vi "FalseTest.vi"() -> ()   [LabVIEW 2016, in "test_AssertControlValue.lvlib"]
uses:
  test_AssertControlValue.lvlib
  main/apis/Setup/GetVI/GetVIByPath.vi
  main/apis/Stimulus/ValueSignal/ValueSignalByPathString.vi
  main/apis/Assert/AssertControlValue/False.vi
  main/apis/Assert/AssertControlValue/Greater.vi
  main/apis/Setup/GetVI/GetVI.lvlib
  <vilib>/addons/_JKI Toolkits/Caraya/classes/Test/Test.lvclass
  main/apis/Assert/AssertControlValue/AssertControlValue.lvlib
panel:
  out "error out":errorcluster
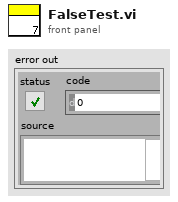
[diagram p1: front panel]
types:
  T1 = enum32{"Invalid", "Standard", "Closed", "Hidden", "Minimized", "Maximized"}
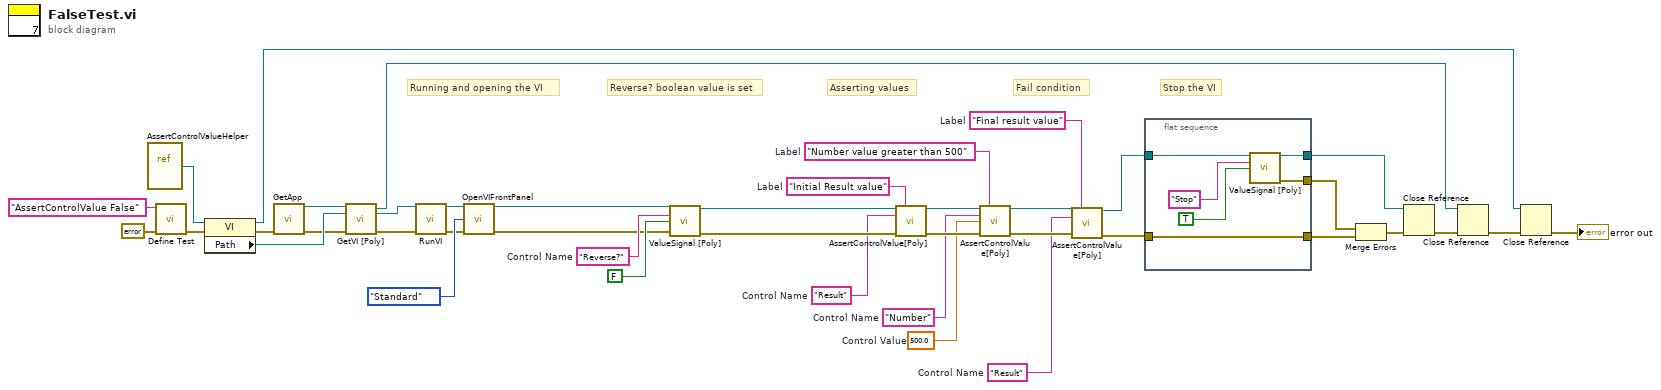
[diagram p0: block diagram]
diagram:
  w5 = "Result"  # Control Name
  w6 = "Final result value"  # Label
  w8 = "Number value greater than 500"  # Label
  w9 = 500.0  # Control Value
  w10 = "Number"  # Control Name
  w16 = "Initial Result value"  # Label
  w27 = "Result"  # Control Name
  w37 = "Reverse?"  # Control Name
  # "Stop the VI"
  # "Asserting values"
  # "Reverse? boolean value is set"
  # "Running and opening the VI"
  # "Fail condition"
  n1 = vi-ref "AssertControlValueHelper.vi"() -> (w31:refnum<vi>)
  n2 = call <vilib>:"Define Test.vi"("error in (no error)"=errorcluster {"status"=FALSE, "code"=0, "source"=""}, "Label (VI Title)"="AssertControlValue False") -> ("error out"=w32:errorcluster)  [unwired: 9 in]
  n3 = property on="Property Node" class="VI"(reference=w31, error in=w32) -> (reference out=w1:refnum<vi>, error out=w40:errorcluster, "Path"=w39:path)
  n4 = call "GetApp.vi"("error in (no error)"=w40) -> ("Application Ref"=w41:refnum<vi>, "error out"=w38:errorcluster)  [unwired: 13 in]
  n5 = call-poly "GetVI [Poly].vi"("Application Ref in"=w41, "VI Path"=w39, "error in (no error)"=w38) -> ("Application Ref out"=w2:refnum<vi>, "VI Reference"=w35:refnum<vi>, "error out"=w34:errorcluster)  [unwired: 10 in]
  n6 = call "RunVI.vi"("VI Reference In"=w35, "error in"=w34) -> ("VI Reference Out"=w17:refnum<vi>, "error out"=w18:errorcluster)  [unwired: 12 in]
  n7 = call "OpenVIFrontPanel.vi"("VI Reference In"=w17, "State(Standard)"=T1."Standard", "error in"=w18) -> ("VI Reference Out"=w21:refnum<vi>, "error out"=w20:errorcluster)  [unwired: 11 in]
  n8 = call-poly "ValueSignal [Poly].vi"("VI Reference In"=w21, "Control Name"=w37, "Value (Signaling)"=FALSE, "error in"=w20) -> ("VI Reference Out"=w28:refnum<vi>, "error out"=w29:errorcluster)  [unwired: 10 in]
  n9 = call-poly "AssertControlValue[Poly].vi"("VI Reference In"=w28, "Label"=w16, "Control Name"=w27, "Error In"=w29) -> ("VI Reference Out"=w12:refnum<vi>, "Error Out"=w14:errorcluster)  [unwired: 10 in]
  n10 = call-poly "AssertControlValue[Poly].vi"("VI Reference In"=w12, "Label"=w8, "Control Name"=w10, "Control Value"=w9, "Error In"=w14) -> ("VI Reference Out"=w11:refnum<vi>, "Error Out"=w15:errorcluster)  [unwired: 9 in]
  n11 = call-poly "AssertControlValue[Poly].vi"("VI Reference In"=w11, "Label"=w6, "Control Name"=w5, "Error In"=w15) -> ("VI Reference Out"=w7:refnum<vi>, "Error Out"=w13:errorcluster)  [unwired: 10 in]
  n12 = flat-sequence {
    tunnel: w7 -> [w45]
    tunnel: [w44] -> w26
    tunnel: w13 -> [w43]
    tunnel: [w43] -> w25
    tunnel: [w42] -> w22
    frame #0 {
      n13 = call-poly "ValueSignal [Poly].vi"("VI Reference In"=w45, "Control Name"="Stop" ("Class Name"), "Value (Signaling)"=TRUE) -> ("VI Reference Out"=w42:refnum<vi>, "error out"=w44:errorcluster)  [unwired: 11 in]
    }
  }
  n14 = Merge Errors(w26, w25) -> (w24:errorcluster)
  n15 = Close Reference(reference=w22, error in (no error)=w24) -> (error out=w23:errorcluster)
  n16 = Close Reference(reference=w2, error in (no error)=w23) -> (error out=w4:errorcluster)
  n17 = Close Reference(reference=w1, error in (no error)=w4) -> (error out=→"error out":errorcluster)
